vi "niScope Fetch From Digitizing Process.vi"(7 "max wait for packet [ms]":i32=50, 8 "error in":errorcluster, 11 "niScope in":T3={"channel cfg"=[], "sessions"=[], "multi cards"=FALSE, "channels"=0, "type"=enum."n/a", "memory [B/chn]"=0, "ext. clock [Hz]"=0.0, "samples count"=0, "use streaming"=FALSE, "proc setup"={"packet size [smpl]"=0, "current timeout [s]"=0.0, "blk2blk timeout [s]"=0.0, "event time"=timestamp(0 s since 1904-01-01), "temp sampl T [s]"=0.0, "data queue"=refnum, "stop notifier"=refnum, "proc ref"=refnum}, "sample width [B]"=0, "ranges [V]"=[], "trigger setup"={"coupling"=1, "level [V]"=0.0, "slope"=0, "mode"=enum."Immediate"}, "fs [Hz]"=0.0, "bitres [bit]"=0} {"trigger setup"."level [V]" format="%.2f"; "trigger setup"."coupling" items=["AC"=0, "DC"=1, "HF Reject"=3, "LF Reject"=4, "AC Plus HF Reject"=1001]; "channel cfg"."Range [Vpk]" min=0.0; "channel cfg"."Channel" min=0}) -> (0 "error out":errorcluster, 1 "auxiliary sampling data":T1, 2 "data block":T2, 3 "niScope out":T3={"channel cfg"=[], "sessions"=[], "multi cards"=FALSE, "channels"=0, "type"=enum."n/a", "memory [B/chn]"=0, "ext. clock [Hz]"=0.0, "samples count"=0, "use streaming"=FALSE, "proc setup"={"packet size [smpl]"=0, "current timeout [s]"=0.0, "blk2blk timeout [s]"=0.0, "event time"=timestamp(0 s since 1904-01-01), "temp sampl T [s]"=0.0, "data queue"=refnum, "stop notifier"=refnum, "proc ref"=refnum}, "sample width [B]"=0, "ranges [V]"=[], "trigger setup"={"coupling"=1, "level [V]"=0.0, "slope"=0, "mode"=enum."Immediate"}, "fs [Hz]"=0.0, "bitres [bit]"=0} {"trigger setup"."level [V]" format="%.2f"; "trigger setup"."coupling" items=["AC"=0, "DC"=1, "HF Reject"=3, "LF Reject"=4, "AC Plus HF Reject"=1001]; "channel cfg"."Range [Vpk]" min=0.0; "channel cfg"."Channel" min=0}, 4 "fetching done?":bool)   [LabVIEW 2018, in "niScope Virtual Digitizer.lvlib"]
doc: "Tries to fetch data block from digitizing data queue. It waits for predefined amount of time. If fetch timeout is reached it returns no data and no error. If digitizing or fetching timeout is reached it returns timout error. If the last data block was detected it also waits for digitizing process exit. If the process won't return it generates error. If the \ndigitizing process terminates prematurely it will return error. The 'auxiliary sampling data' are valid only if 'valid?' flag in it is True. 'Data block' content is valid only if 'valid?' flag is true. The caller of this VI must collect the data whenever the 'valid?' flag(s) are True. Caller of this VI must always check 'fetching done?' flag and when it is True or function returned error it shall not be called again."
uses:
  niScope Virtual Digitizer.lvlib
  niScope Session.ctl
  niScope Virtual Channel Config.ctl
  niScope Virtual Channel Mode.ctl
  niScope Virtual Channel Input Z.ctl
  niScope Virtual Channel Coupling.ctl
  niScope Type.ctl
  niScope Digitizing Process Options.ctl
  niScope Data Packet.ctl
  niScope Trigger Setup.ctl
  <instrlib>/niScope/Controls/niScope trigger coupling.ctl
  <instrlib>/niScope/Controls/niScope trigger slope.ctl
  niScope Record Aux Data.ctl
  <vilib>/Utility/error.llb/Error Cluster From Error Code.vi
  <vilib>/ErrorRing/Error Ring.xnode
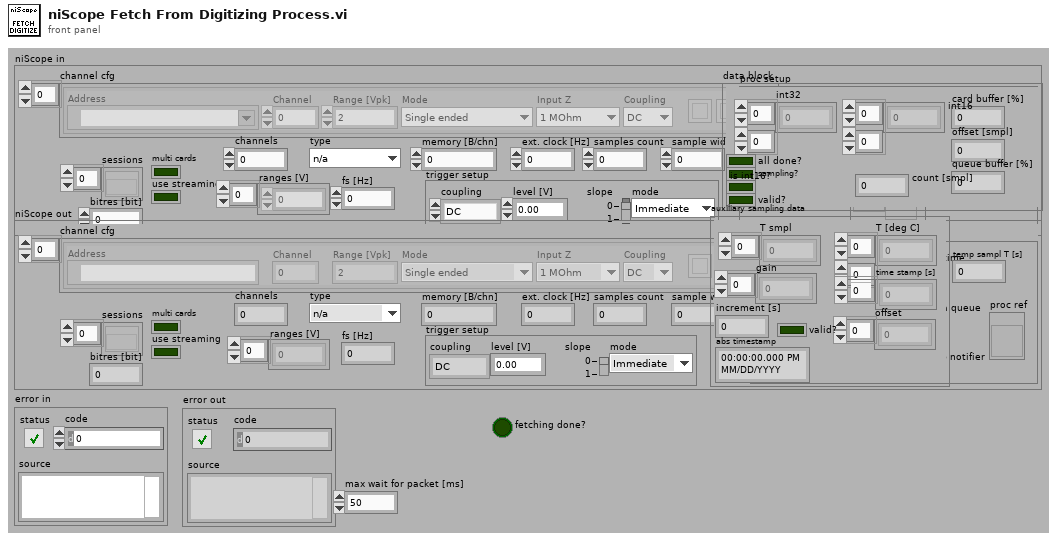
[diagram p1: front panel]
types:
  T1 = typedef "niScope Virtual Digitizer.lvlib/niScope Record Aux Data.ctl" = cluster{"T smpl":i64[], "T [deg C]":dbl[][], "time stamp [s]":dbl[], "offset":dbl[], "gain":dbl[], "increment [s]":dbl, "valid?":bool, "abs timestamp":timestamp}
  T2 = typedef "niScope Virtual Digitizer.lvlib/niScope Data Packet.ctl" = cluster{"int32":i32[][], "card buffer [%]":dbl, "all done?":bool, "offset [smpl]":i64, "sampling?":bool, "queue buffer [%]":dbl, "int16":i16[][], "is int16?":bool, "count [smpl]":i32, "valid?":bool}
  T3 = typedef "niScope Virtual Digitizer.lvlib/niScope Session.ctl" = cluster{"channel cfg":T4[], "sessions":refnum<k20>[], "multi cards":bool, "channels":i32, "type":T8, "memory [B/chn]":i32, "ext. clock [Hz]":dbl, "samples count":i64, "use streaming":bool, "proc setup":T9, "sample width [B]":i32, "ranges [V]":dbl[], "trigger setup":T10, "fs [Hz]":dbl, "bitres [bit]":i32}
  T4 = typedef "niScope Virtual Digitizer.lvlib/niScope Virtual Channel Config.ctl" = cluster{"Address":refnum<k15>, "Channel":i32, "Mode":T5, "Input Z":T6, "Coupling":T7, "Range [Vpk]":dbl, "btn clr":bool, "btn up":bool, "btn down":bool}
  T5 = typedef "niScope Virtual Digitizer.lvlib/niScope Virtual Channel Mode.ctl" = enum16{"Single ended", "Unbal. differential", "Differential"}
  T6 = typedef "niScope Virtual Digitizer.lvlib/niScope Virtual Channel Input Z.ctl" = enum16{"1 MOhm", "50 Ohm"}
  T7 = typedef "niScope Virtual Digitizer.lvlib/niScope Virtual Channel Coupling.ctl" = enum16{"AC", "DC", "GND"}
  T8 = typedef "niScope Virtual Digitizer.lvlib/niScope Type.ctl" = enum16{"n/a", "5922"}
  T9 = typedef "niScope Virtual Digitizer.lvlib/niScope Digitizing Process Options.ctl" = cluster{"packet size [smpl]":i64, "current timeout [s]":dbl, "blk2blk timeout [s]":dbl, "event time":timestamp, "temp sampl T [s]":dbl, "data queue":refnum<queue>, "stop notifier":refnum<notifier>, "proc ref":refnum<vi>}
  T10 = typedef "niScope Virtual Digitizer.lvlib/niScope Trigger Setup.ctl" = cluster{"coupling":T11, "level [V]":dbl, "slope":T12, "mode":enum16{"Immediate", "External", "Level"}}
  T11 = typedef "niScope trigger coupling.ctl" = u16
  T12 = typedef "niScope trigger slope.ctl" = i32
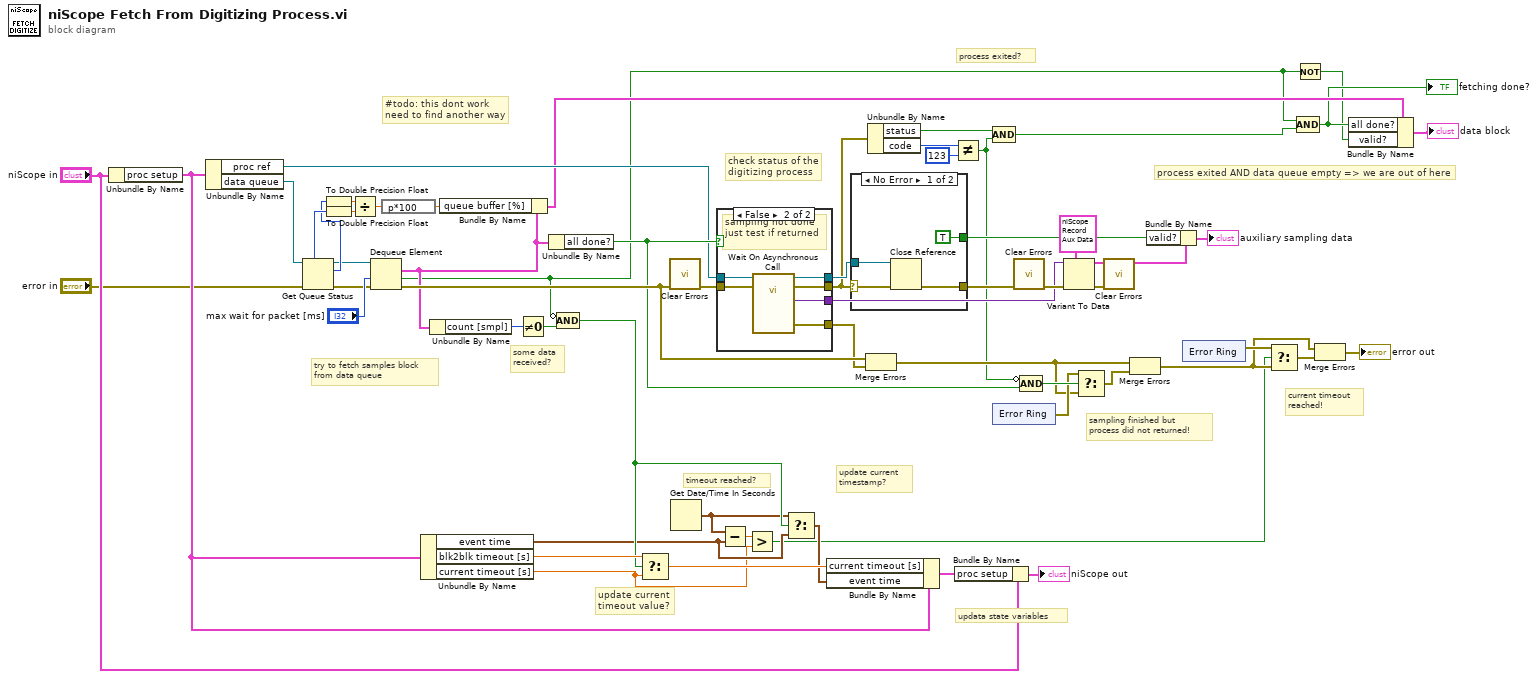
[diagram p0: block diagram]
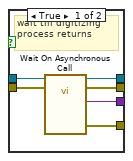
[diagram p3: hidden frame]
diagram:
  # "process exited AND data queue empty => we are out of here"
  # "process exited?"
  # "update current\ntimestamp?"
  # "update current \ntimeout value?"
  # "some data\nreceived?"
  # "#todo: this dont work\nneed to find another way"
  # "updata state variables"
  # "check status of the\ndigitizing process"
  # "try to fetch samples block\nfrom data queue"
  # "current timeout\nreached!"
  # "sampling finished but\nprocess did not returned!"
  # "timeout reached?"
  n1 = Unbundle By Name("niScope in") -> ("proc setup"=w41:T9)
  n2 = Unbundle By Name(w41) -> ("proc ref"=w42:refnum<vi>, "data queue"=w29:refnum<queue>)
  n3 = Get Queue Status(queue=w29, error in (no error)="error in") -> (queue out=w31:refnum<queue>, max queue size=w37:i32, # pending remove=w32:i32, error out=w38:errorcluster)  [unwired: 1 in, 4 out]
  n4 = To Double Precision Float(number=w32) -> (double precision float=w33:dbl)
  n5 = To Double Precision Float(number=w37) -> (double precision float=w34:dbl)
  n6 = Divide(x=w33, y=w34) -> (x/y=w36:dbl)
  n7 = Dequeue Element(queue=w31, timeout in ms (-1)="max wait for packet [ms]", error in (no error)=w38) -> (element=w25:T2, timed out?=w1:bool, error out=w57:errorcluster)  [unwired: 1 out]
  n8 = expression code="p*100"(w36) -> (w35:dbl)
  n9 = Unbundle By Name(w41) -> ("event time"=w19:timestamp, "blk2blk timeout [s]"=w22:dbl, "current timeout [s]"=w4:dbl)
  n10 = Unbundle By Name(w25) -> ("count [smpl]"=w24:i32)
  n11 = Bundle By Name(cluster=w25, "queue buffer [%]"=w35) -> (w26:T2)
  n12 = Not Equal To 0?(x=w24) -> (x != 0?=w23:bool)
  n13 = Unbundle By Name(w25) -> ("all done?"=w49:bool)
  n14 = Compound Arithmetic op=AND(invert w1, w23) -> (w21:bool)
  n15 = Select(t=w22, s=w21, f=w4) -> (s? t:f=w18:dbl)
  n16 = call <vilib>:"Clear Errors.vi"("error in (no error)"=w57) -> ("error out"=w58:errorcluster)  [unwired: 5 in, 1 out]
  n17 = Get Date/Time In Seconds() -> (seconds since 1Jan1904=w20:timestamp)
  n18 = case shown="False" w49 {
    tunnel: w42 -> [w66 w72]
    tunnel: w58 -> [w65 w71]
    tunnel: [w64 w70] -> w56
    tunnel: [w63 w69] -> w10
    tunnel: [w62 w68] -> w12
    tunnel: [w61 w67] -> w43
    frame True {
      # "wait till digitizing\nprocess returns"
      n19 = call-by-ref "Wait On Asynchronous Call"(reference=w66, error in=w65) -> (reference out=w61:refnum<vi>, error out=w63:errorcluster, 0:"error out"=w64:errorcluster, "auxiliary data out"=w62:variant)  [unwired: 10 in]
    }
    frame False {
      # "sampling not done\njust test if returned"
      n20 = call-by-ref "Wait On Asynchronous Call"(reference=w72, error in=w71) -> (reference out=w67:refnum<vi>, error out=w69:errorcluster, 0:"error out"=w70:errorcluster, "auxiliary data out"=w68:variant)  [unwired: 10 in]
    }
  }
  n21 = Subtract(x=w20, y=w19) -> (x-y=w59:dbl)
  n22 = Greater?(x=w59, y=w4) -> (0:w16:bool)
  n23 = Select(t=w20, s=w21, f=w19) -> (s? t:f=w17:timestamp)
  n24 = Bundle By Name(cluster=w41, "current timeout [s]"=w18, "event time"=w17) -> (w40:T9)
  n25 = case shown="No Error" w10 {
    selector: w10 -> [w76 w77]
    tunnel: [w75 w77] -> w44
    tunnel: w43 -> [w74 _]
    tunnel: [TRUE _] -> w11
    frame No Error {
      n26 = Close Reference(reference=w74, error in (no error)=w76) -> (error out=w75:errorcluster)
    }
    frame Error {
      # "timeout or\nalready eaxited"
    }
  }
  n27 = Merge Errors(w57, w56) -> (w52:errorcluster)
  n28 = Unbundle By Name(w10) -> ("status"=w7:bool, "code"=w9:i32)
  n29 = Not Equal?(x=w9, y=123) -> (x != y?=w3:bool)
  n30 = Bundle By Name(cluster="niScope in", "proc setup"=w40) -> (→"niScope out":T3)
  n31 = Compound Arithmetic op=AND(w7, w3) -> (w2:bool)
  n32 = xnode "Error Ring"() -> ("error out"=w53:errorcluster)
  n33 = call <vilib>:"Clear Errors.vi"("error in (no error)"=w44) -> ("error out"=w50:errorcluster)  [unwired: 5 in, 1 out]
  n34 = Compound Arithmetic op=AND(invert w3, w49) -> (w54:bool)
  n35 = Variant To Data(error in=w50, type=T1 {"T smpl"=[], "T [deg C]"=[], "time stamp [s]"=[], "offset"=[], "gain"=[], "increment [s]"=0.0, "valid?"=FALSE, "abs timestamp"=timestamp(0 s since 1904-01-01)} ("aux data"), Variant=w12) -> (data=w14:T1, error out=w13:errorcluster)
  n36 = Select(t=w53, s=w54, f=w52) -> (s? t:f=w51:errorcluster)
  n37 = call <vilib>:"Clear Errors.vi"("error in (no error)"=w13) -> ()  [unwired: 5 in, 2 out]
  n38 = Merge Errors(w52, w51) -> (w46:errorcluster)
  n39 = Bundle By Name(cluster=w14, "valid?"=w11) -> (→"auxiliary sampling data":T1)
  n40 = xnode "Error Ring"() -> ("error out"=w48:errorcluster)
  n41 = Select(t=w48, s=w16, f=w46) -> (s? t:f=w47:errorcluster)
  n42 = Not(x=w1) -> (.not. x?=w5:bool)
  n43 = Compound Arithmetic op=AND(w1, w2) -> (w6:bool)
  "fetching done?" <- w6
  n44 = Merge Errors(w46, w47) -> (→"error out":errorcluster)
  n45 = Bundle By Name(cluster=w26, "all done?"=w6, "valid?"=w5) -> (→"data block":T2)
